vi "teststreamer nowait server.vi"() -> ()   [LabVIEW 2016]
uses:
  dllwrapper/action complete event.ctl
  tls classes/connection creator/server acceptor/server acceptor.lvclass
  C:/Users/IEUser/Desktop/libasynclvtls/tls classes/connection creator/connection creator.lvclass
  tls classes/engine context/engine context.lvclass
  tls classes/connection/connection.lvclass
  tls classes/connection creator/connection creator.lvclass
  dllwrapper/async tls dl.lvlib
  <vilib>/ptbypt/NI_PtbyPt.lvlib
panel:
  out "Numeric":dbl
  out "Waveform Chart":dbl(graph)
  out "bytes/s":dbl format="%#_9g"
  out "bytes written":i32
  in  "stop":bool
  out "error out 3":errorcluster
  out "error out 2":errorcluster
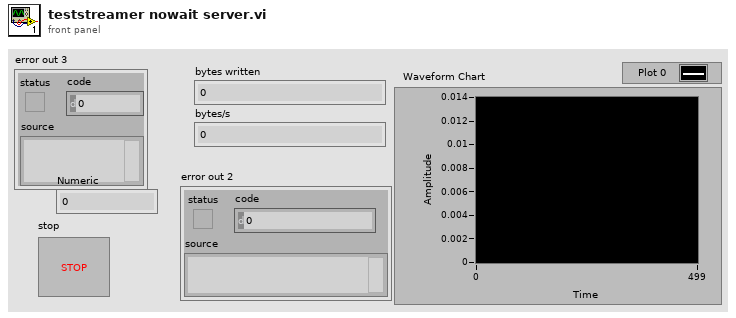
[diagram p1: front panel]
types:
  T1 = typedef "async tls dl.lvlib/action complete event.ctl" = cluster{"request ID":u32, "error code":i32, "error string":string}
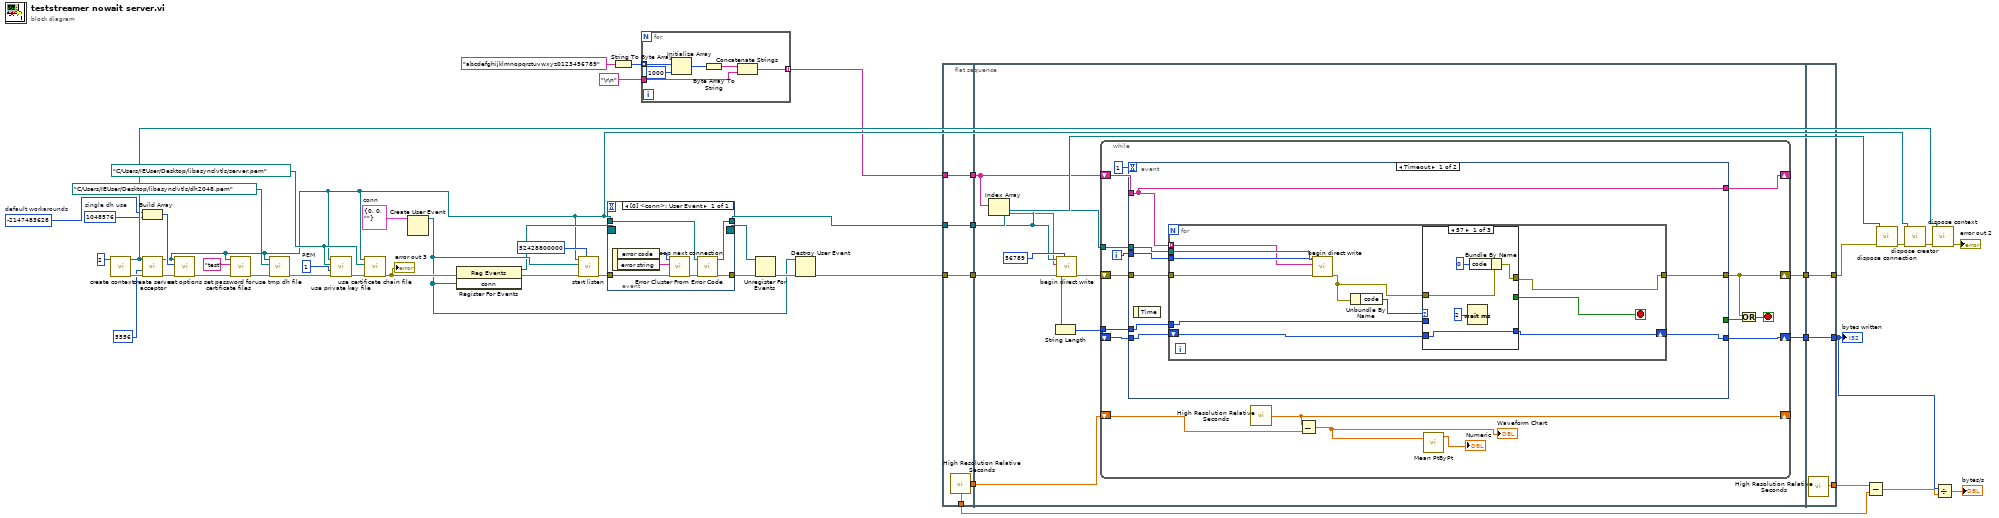
[diagram p0: block diagram]
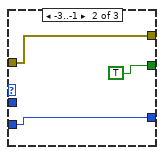
[diagram p2: hidden frame]
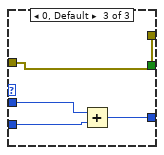
[diagram p3: hidden frame]
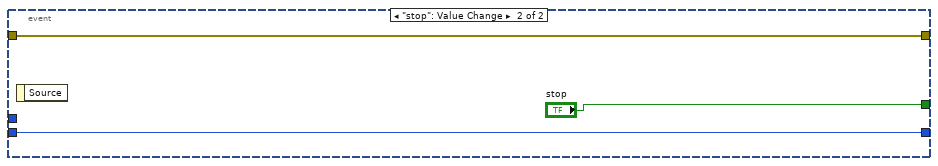
[diagram p4: hidden frame]
diagram:
  w28 = T1 {"request ID"=0, "error code"=0, "error string"=""}  # conn
  w33 = 1  # PEM
  w38 = path "C:/Users/IEUser/Desktop/libasynclvtls/server.pem" ("cert chain file")
  w41 = -2147483628  # default workarounds
  w42 = 1048576  # single dh use
  n1 = call "create context.vi"("thread count"=u64 2) -> ("error out"=w45:errorcluster, "engine context out"=w44:refnum<class "engine context.lvclass">)  [unwired: 9 in]
  n2 = Build Array(w41, w42) -> (w35:i32[])
  n3 = call "create server acceptor.vi"("error in"=w45, "port"=u16 5556, "engine context in"=w44) -> ("error out"=w43:errorcluster, "server acceptor out"=w18:refnum<class "server acceptor.lvclass">)  [unwired: 7 in]
  n4 = call "set options.vi"("error in"=w43, "options"=w35, "connection creator in"=w18) -> ("error out"=w40:errorcluster)  [unwired: 8 in]
  n5 = call "set password for certificate files.vi"("error in"=w40, "password"="test" ("file"), "connection creator in"=w18) -> ("error out"=w32:errorcluster)  [unwired: 8 in]
  n6 = call "use tmp dh file.vi"("error in"=w32, "tmp dh file"=path "C:/Users/IEUser/Desktop/libasynclvtls/dh2048.pem", "connection creator in"=w18) -> ("error out"=w31:errorcluster)  [unwired: 8 in]
  n7 = call "use private key file.vi"("error in"=w31, "format"=w33, "private key file"=w38, "connection creator in"=w18) -> ("error out"=w30:errorcluster)  [unwired: 7 in]
  n8 = call "use certificate chain file.vi"("error in"=w30, "cert chain file"=w38, "connection creator in"=w18) -> ("error out"=w37:errorcluster)  [unwired: 8 in]
  "error out 3" <- w37
  n9 = Create User Event(user event datatype=w28) -> (user event=w24:refnum<user-event>)  [unwired: 1 in, 1 out]
  n10 = register-events(error in=w37, w24) -> (reference out=w20:refnum<event-registration>, error out=w27:errorcluster)  [unwired: 1 in]
  n11 = call "start listen.vi"("stream buffer size"=u64 52428800000, "error in"=w27, "completion event"=w24, "server acceptor in"=w18) -> ("error out"=w22:errorcluster)  [unwired: 7 in]
  n12 = event shown="[0] <conn>: User Event" {
    selector: w20 -> [_]
    dyn-events: [_] -> w21
    timeout: _ -> [_]
    tunnel: [w54] -> w23
    tunnel: w22 -> [w55]
    tunnel: w18 -> [w50]
    tunnel: [w49] -> w17
    event User Event {
      n13 = event-data() -> ("error code"=w52:i32, "error string"=w51:string)  [unwired: 1 in]
      n14 = call <vilib>:"Error Cluster From Error Code.vi"("error in (no error)"=w55, "error message (\"\")"=w51, "error code (0)"=w52) -> ("error out"=w53:errorcluster)  [unwired: 6 in]
      n15 = call "pop next connection.vi"("error in"=w53, "connection creator in"=w50) -> ("error out"=w54:errorcluster, "connection out"=w49:refnum<class "connection.lvclass">)  [unwired: 8 in]
    }
  }
  n16 = String To Byte Array(string="abcdefghijklmnopqrstuvwxyz0123456789") -> (unsigned byte array=w16:u8[])
  n17 = for {
    tunnel: w16 -> [w61] mode=indexing
    tunnel: [w58] -> w1 mode=indexing
    tunnel: "\r\n" ("termination") -> [w57]
    n18 = Initialize Array(w61, 1000 ("dimension size")) -> (w60:u8[])
    n19 = Byte Array To String(unsigned byte array=w60) -> (string=w59:string)
    n20 = Concatenate Strings(w59, w57) -> (w58:string)
  }
  n21 = Unregister For Events(event registration refnum=w21, error in=w23) -> (error out=w26:errorcluster)
  n22 = Destroy User Event(user event=w24, error in=w26) -> (error out=w25:errorcluster)
  n23 = flat-sequence {
    tunnel: w1 -> [w63]
    tunnel: w17 -> [w64]
    tunnel: w25 -> [w65]
    tunnel: [w65] -> w13
    tunnel: [w64] -> w12
    tunnel: [w63] -> w11
    tunnel: [w62] -> w8
    tunnel: [w62] -> w2
    tunnel: w13 -> [w73]
    tunnel: w12 -> [w71]
    tunnel: w11 -> [w70]
    tunnel: [w72] -> w10
    tunnel: [w67] -> w7
    tunnel: w2 -> [w66]
    tunnel: [w128] -> w19
    tunnel: w10 -> [w128]
    tunnel: [w127] -> w9
    tunnel: [w126] -> w5
    tunnel: w7 -> [w126]
    frame #0 {
      n24 = call <vilib>:"High Resolution Relative Seconds.vi"() -> ("relative seconds"=w62:dbl)
    }
    frame #1 {
      n25 = Index Array(array=w70) -> (element=w69:string)  [unwired: 1 in]
      n26 = String Length(string=w69) -> (length=w68:i32)
      n27 = call "begin direct write.vi"("id"=u32 56789, "error in"=w73, "data"=w69, "connection in"=w71) -> ("error out"=w74:errorcluster)  [unwired: 6 in, 1 out]
      n28 = while {
        shift-right: [w88] -> w72
        shift-left: w74 -> [w91]
        tunnel: w71 -> [w90]
        shift-right: [w85] -> _
        shift-left: w70 -> [w86]
        tunnel: w68 -> [w83]
        shift-right: [w82] -> w67
        shift-left: w68 -> [w81]
        shift-right: [w79] -> _
        shift-left: w66 -> [w80]
        i -> [w84]
        stop <- w89 stop-if-true
        n29 = event shown="[0] Timeout" {
          selector: _ -> [_ _]
          dyn-events: _ -> [_ _]
          timeout: 1 -> [_ _]
          tunnel: w91 -> [w99 w124]
          tunnel: w90 -> [w97 _]
          tunnel: [w98 w124] -> w88
          tunnel: [_ "stop"] -> w87
          tunnel: w86 -> [w92 _]
          tunnel: [w92 _] -> w85
          tunnel: w84 -> [w96 _]
          tunnel: w83 -> [w93 _]
          tunnel: [w95 w123] -> w82
          tunnel: w81 -> [w94 w123]
          event Timeout {
            n30 = event-data() -> ()  [unwired: 1 in, 1 out]
            n31 = for {
              tunnel: w97 -> [w109]
              tunnel: w96 -> [w108]
              tunnel: w93 -> [w105]
              shift-right: [w107] -> w95
              shift-left: w94 -> [w106]
              tunnel: w92 -> [w104] mode=indexing
              tunnel: w99 -> [w110]
              tunnel: [w101] -> w98
              stop <- w102 stop-if-true
              n32 = call "begin direct write.vi"("id"=w108, "error in"=w110, "data"=w104, "connection in"=w109) -> ("error out"=w100:errorcluster)  [unwired: 6 in, 1 out]
              n33 = Unbundle By Name(w100) -> ("code"=w103:i32)
              n34 = case shown="57" w103 {
                tunnel: [w115 w118 w122] -> w107
                tunnel: w106 -> [w115 w118 w121]
                tunnel: w105 -> [_ _ w120]
                tunnel: [_ TRUE _] -> w102
                tunnel: [w112 w116 w119] -> w101
                tunnel: w100 -> [w113 w116 w119]
                frame 57 {
                  n35 = Wait (ms)(milliseconds to wait=u32 2) -> ()  [unwired: 1 out]
                  n36 = Bundle By Name(cluster=w113, "code"=0) -> (w112:errorcluster)
                }
                frame -3..-1 {
                }
                frame 0, Default {
                  n37 = Add(x=w120, y=w121) -> (x+y=w122:i32)
                }
              }
            }
          }
          event "stop": Value Change {
            n38 = event-data() -> ()  [unwired: 1 in, 1 out]
          }
        }
        n39 = call <vilib>:"High Resolution Relative Seconds.vi"() -> ("relative seconds"=w79:dbl)
        n40 = Subtract(x=w79, y=w80) -> (x-y=w77:dbl)
        "Waveform Chart" <- w77
        n41 = call <vilib>:"Mean PtByPt.vi"("x"=w77) -> ("mean"=→"Numeric":dbl)  [unwired: 3 in, 1 out]
        n42 = Or(x=w88, y=w87) -> (x .or. y?=w89:bool)
      }
    }
    frame #2 {
      n43 = call <vilib>:"High Resolution Relative Seconds.vi"() -> ("relative seconds"=w127:dbl)
    }
  }
  n44 = Subtract(x=w9, y=w8) -> (x-y=w6:dbl)
  n45 = call "dispose connection.vi"("error in"=w19, "connection in"=w17) -> ("error out"=w48:errorcluster)  [unwired: 9 in]
  n46 = call "dispose creator.vi"("error in"=w48, "connection creator in"=w18) -> ("error out"=w47:errorcluster)  [unwired: 9 in]
  n47 = call "dispose context.vi"("error in"=w47, "engine context out"=w44) -> ("error out"=→"error out 2":errorcluster)  [unwired: 9 in]
  n48 = Divide(x=w5, y=w6) -> (x/y=→"bytes/s":dbl)
  "bytes written" <- w5
